vi "FPGA Main with speed output.vi"() -> ()   [LabVIEW 2018]
doc: "This VI reads all analogue data channels available at the fastest rate supported by the respective hardware and updates a memory address for when each measurement is available.\n\nAt a rate defined by the fastest module (NI 9237 - default of 12.5kHz) this memory is read, combined with the measurements from the 9237 module and written to the FIFO for communication to the RT machine.\n\nThe NI 9237 modeul therefore defines the nominal sampling rate of the system (with slower channels over-sampled).\n\nA time channel (in uSec) is provided with 0 referenced from the first acquisition of the NI 9237 module"
uses:
  <vilib>/LabVIEW Targets/FPGA/cRIO/shared/nicrio_ModuleControls/nicrio_cRIO-9237_DataRatesRing.ctl
  <vilib>/Platform/TimedLoop/XDataNode/timing_clust.ctl
  <vilib>/Platform/TimedLoop/XDataNode/nitl_modes.ctl
  <vilib>/Platform/TimedLoop/XDataNode/wakeup.ctl
  <vilib>/rvi/Emulation/niFpgaGetClockAttributes.vi
  <vilib>/rvi/Emulation/niFpgaSctlEmulationGetInTimedLoop.vi
  <vilib>/rvi/Emulation/niFpgaEmulationReportErrorSimple.vi
  <vilib>/rvi/Emulation/niFpgaProcessEmulError.vi
  <vilib>/rvi/eio/common/nirviEmuTemplatePropertySet_noerrors.vi
  <vilib>/rvi/eio/common/nirviEmuTemplateMethod_errors.vi
  <vilib>/rvi/interface/RandomDataEmulation/niFpgaRandomDataHandleErrors.vi
  <vilib>/rvi/Memory/Memory_Emulation/nirvimemoryFastEmulation.vi
  <vilib>/rvi/Memory/Memory_Emulation/nirvimemoryEmulation.vi
  <vilib>/rvi/Emulation/niFpgaEmulationIsFPGAContextNoSignature.vi
  <vilib>/rvi/DataTransferAndStorage/Container/Common/niFpgaContainerGetUniqueNameForEmu.vi
  <vilib>/rvi/errors/nirviReportUnexpectedCaseInternalError (U32).vi
  <vilib>/rvi/Emulation/niFpgaCriticalErrorInLSC.vi
  <vilib>/eio/EIOPropertyNode/EIOPropertyNode.xnode
  <vilib>/eio/EIONode/EIONode.xnode
  <vilib>/rvi/DataTransferAndStorage/Container/XNode/niFpgaContainer.xnode
  <vilib>/rvi/interface/RandomDataEmulation/nirviRandomDataFpgaReadWriteTemplate.vi
  <vilib>/platform/TimedLoop/XDataNode/XDataNode.xnode
  <vilib>/eio/EIOMethodNode/EIOMethodNode.xnode
  <vilib>/Platform/TimedLoop/XDataNode/XDNodeRunTimeDep.lvlib
  <vilib>/rvi/eio/common/nirviEmuTemplatePropertyGet_errors.vi
  <vilib>/rvi/eio/common/nirviEmuTemplatePropertyGet_noerrors.vi
  <vilib>/rvi/eio/common/nirviEmuTemplatePropertySet_errors.vi
panel:
  in  "speedOutputScaling":sgl=6366198.0
  in  "speedDirection":bool=TRUE
  in  "speed filter":u16=150
  in  "switch encoders":bool
  in  "falling edge (F)":bool caption="Torque encoder direction"
  in  "filterTorque":bool
  in  "Data Rate":T1=1 items=["50.000 kS/s (NI 9237)"=1, "25.000 kS/s (NI 9237)"=2, "16.667 kS/s (NI 9237)"=3, "12.500 kS/s (NI 9237)"=4, "10.000 kS/s (NI 9237)"=5, "8.333 kS/s (NI 9237)"=6, "7.143 kS/s (NI 9237)"=7, "6.250 kS/s (NI 9237)"=8, "5.556 kS/s (NI 9237)"=9, "5.000 kS/s (NI 9237)"=10, "4.545 kS/s (NI 9237)"=11, "4.167 kS/s (NI 9237)"=12, "3.846 kS/s (NI 9237)"=13, "3.571 kS/s (NI 9237)"=14, "3.333 kS/s (NI 9237)"=15, "3.125 kS/s (NI 9237)"=16, "2.941 kS/s (NI 9237)"=17, "2.778 kS/s (NI 9237)"=18, "2.632 kS/s (NI 9237)"=19, "2.500 kS/s (NI 9237)"=20, "2.381 kS/s (NI 9237)"=21, "2.273 kS/s (NI 9237)"=22, "2.174 kS/s (NI 9237)"=23, "2.083 kS/s (NI 9237)"=24, "2.000 kS/s (NI 9237)"=25, "1.923 kS/s (NI 9237)"=26, "1.852 kS/s (NI 9237)"=27, "1.786 kS/s (NI 9237)"=28, "1.724 kS/s (NI 9237)"=29, "1.667 kS/s (NI 9237)"=30, "1.613 kS/s (NI 9237)"=31]
  in  "encoders offset":sgl caption="encoder offset (radians)"
  out "Total channel count":u32=61
  out "timestamp":u32
  out "FIFO full counter":i32
  in  "Safe Voltage":fxp<+/-,20,5>[](array[numeric])=[0.0, 0.0, 0.0, 0.0]
  in  "Safe Digital":bool[](array[boolean])=[FALSE, FALSE, FALSE, FALSE, FALSE, FALSE, FALSE, FALSE]
  in  "Voltage Out":fxp<+/-,20,5>[](array[numeric])=[0.0, 0.0, 0.0, 0.0]
  in  "Update Outputs":bool
  in  "Mod 8":bool[](array[boolean])=[FALSE, FALSE, FALSE, FALSE, FALSE, FALSE, FALSE, FALSE]
  out "E Stop":bool
  in  "Stop acquire":bool
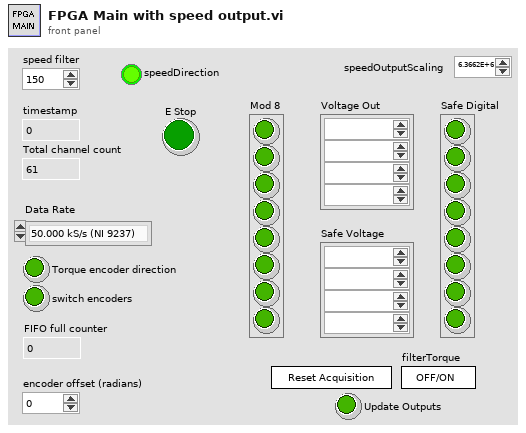
[diagram p1: front panel]
types:
  T1 = typedef "nicrio_cRIO-9237_DataRatesRing.ctl" = u8
  T2 = typedef "XDNodeRunTimeDep.lvlib/timing_clust.ctl" = cluster{"Expected End [f-1]":u64, "Actual End [f-1]":u64, "Finished Late? [f-1]":bool, "Expected End [i-1]":u64, "Actual End [i-1]":u64, "Finished Late? [i-1]":bool, "Expected Start [i]":u64, "Actual Start [i]":u64, "Expected Start [f]":u64, "Actual Start [f]":u64, "Source Name":string, "Structure Name":string, "Period":i64, "Deadline":i64, "Offset":i64, "Start":i64, "Priority":i32, "Timeout":i32, "Mode":T3, "Wakeup Reason":T4, "Error":errorcluster, "Source Type":string, "Secondary Source Type":string, "Global End Time":u64, "Global Start Time":u64, "Frame Duration":u64, "Iteration Duration":u64, "Assigned CPU":i32, "I/O Scan Engine Mode":u32}
  T3 = typedef "XDNodeRunTimeDep.lvlib/nitl_modes.ctl" = enum32{"No Change", "Process missed periods, maintain original phase", "Discard missed periods, maintain original phase", "Process missed periods, ignore original phase", "Discard missed periods, ignore original phase"}
  T4 = typedef "XDNodeRunTimeDep.lvlib/wakeup.ctl" = enum32{"Normal", "Aborted", "Asynchronous wakeup", "Timing source error", "Timed loop error", "Timeout"}
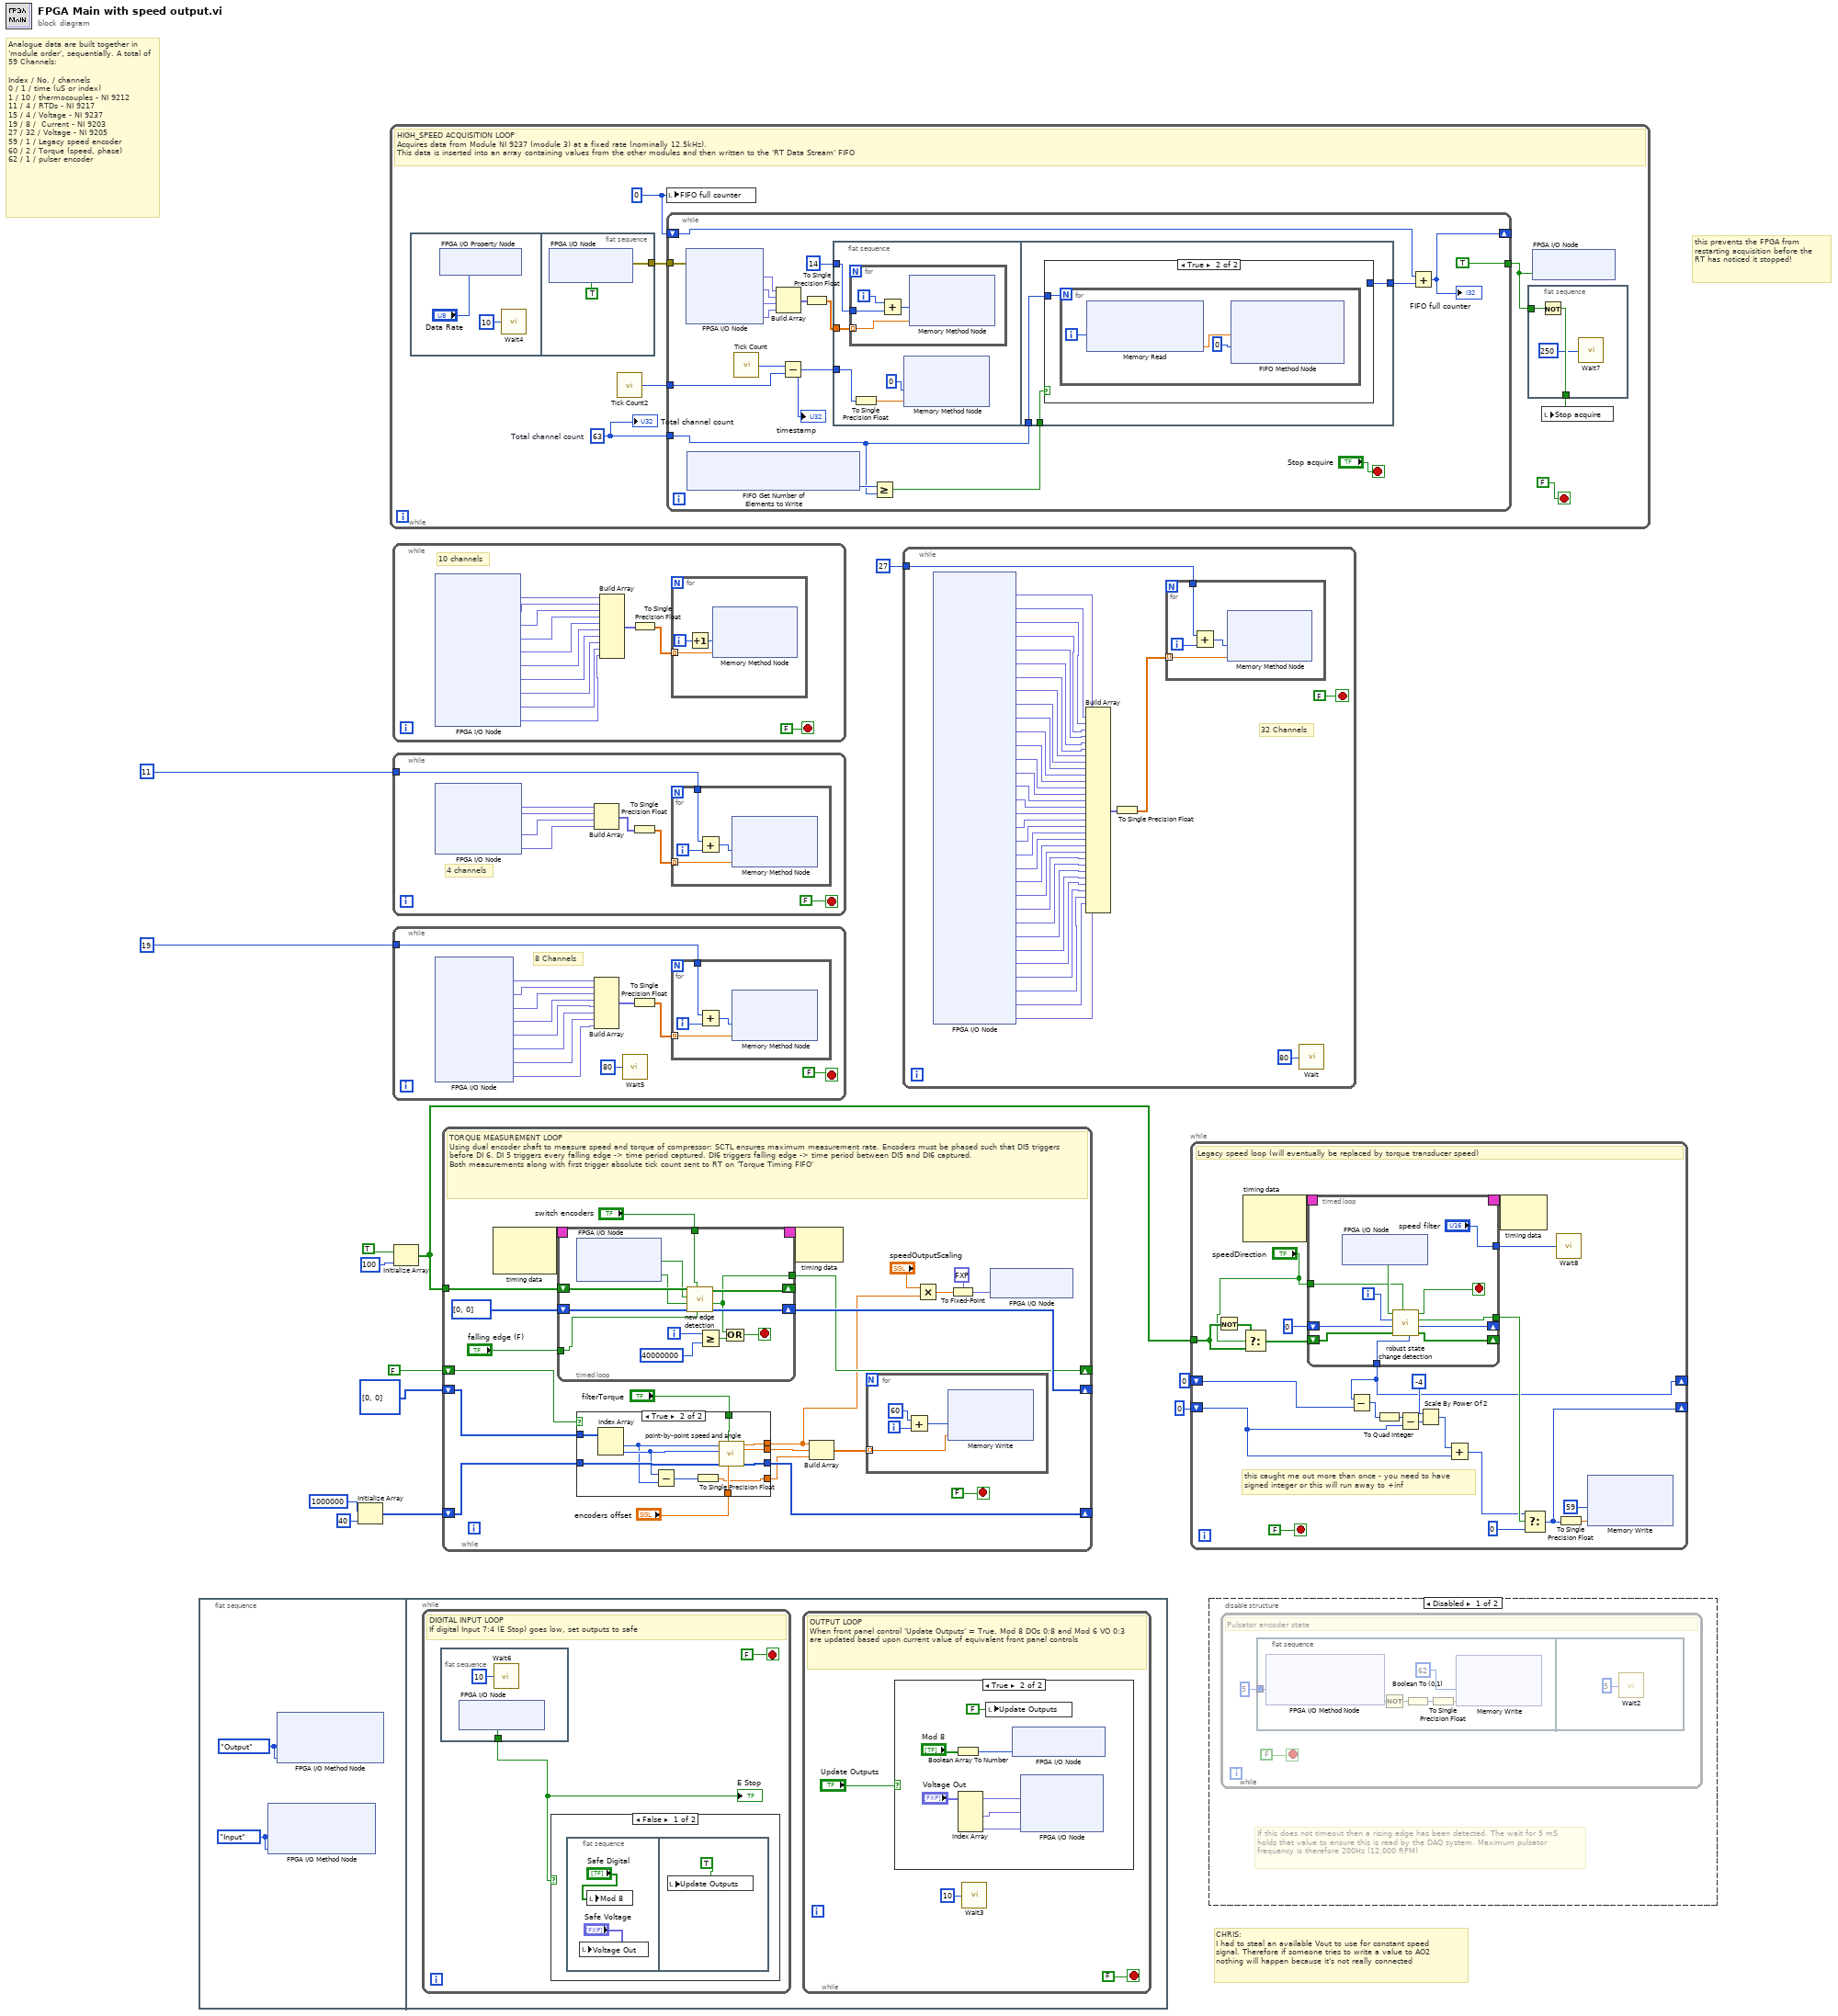
[diagram p0: block diagram]
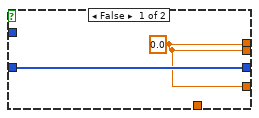
[diagram p5: hidden frame]
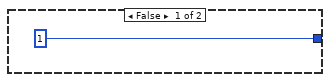
[diagram p6: hidden frame]
diagram:
  # "CHRIS:\nI had to steal an available Vout to use for constant speed signal. Therefore if someone tries to write a value to AO2 nothing will happen because it's not really connected"
  # "this prevents the FPGA from restarting acquisition before the RT has noticed it stopped!"
  # "Analogue data are built together in 'module order', sequentially. A total of 59 Channels:\n\nIndex / No. / channels\n0 / 1 / time (uS or index)\n1 / 10 / thermocouples - NI 9212\n11 / 4 / RTDs - NI 9217\n15 / 4 / Voltage - NI 9237\n19 / 8 /  Current - NI 9203\n27 / 32 / Voltage - NI 9205\n59 / 1 / Legacy speed encoder\n60 / 2 / Torque (speed, phase)\n62 / 1 / pulser encoder"
  n1 = flat-sequence {
    frame #0 {
      w14 = enum8{"No Change", "Input", "Output"}."Output" ("DIO 7:4")
      w15 = enum8{"No Change", "Input", "Output"}."Input" ("DIO 7:4")
      n2 = xnode "FPGA I/O Method Node"("DIO 7:4"=w15, "DIO 3:0"=w15) -> ()  [unwired: 1 in, 1 out]
      n3 = xnode "FPGA I/O Method Node"("DIO 7:4"=w14, "DIO 3:0"=w14) -> ()  [unwired: 1 in, 1 out]
    }
    frame #1 {
      n4 = while {
        stop <- FALSE stop-if-true
        # "DIGITAL INPUT LOOP\nIf digital Input 7:4 (E Stop) goes low, set outputs to safe"
        n5 = flat-sequence {
          tunnel: [w29] -> w26
          frame #0 {
            n6 = xnode "FPGA I/O Node"() -> ("Mod7/DIO4"=w29:bool)  [unwired: 1 in, 1 out]
            n7 = call "Wait6"("Count(uSec)"=u8 10) -> ()  [unwired: 1 out]
          }
        }
        n8 = case shown="False" w26 {
          frame False {
            n9 = flat-sequence {
              frame #0 {
                n10 = local write "Voltage Out"("Safe Voltage") -> ()
                n11 = local write "Mod 8"("Safe Digital") -> ()
              }
              frame #1 {
                n12 = local write "Update Outputs"(TRUE ("Update Outputs")) -> ()
              }
            }
          }
          frame True {
          }
        }
        "E Stop" <- w26
      }
      n13 = while {
        stop <- FALSE stop-if-true
        # "OUTPUT LOOP\nWhen front panel control 'Update Outputs' = True, Mod 8 DOs 0:8 and Mod 6 VO 0:3 are updated based upon current value of equivalent front panel controls"
        n14 = case shown="True" "Update Outputs" {
          frame False {
          }
          frame True {
            n15 = Boolean Array To Number(Boolean array="Mod 8") -> (number=w24:u8)
            n16 = Index Array(array="Voltage Out") -> (element #1=w22:fxp<+/-,20,5>, element #2=w21:fxp<+/-,20,5>, element #4=w19:fxp<+/-,20,5>)  [unwired: 4 in, 1 out]
            n17 = local write "Update Outputs"(FALSE ("Update Outputs")) -> ()
            n18 = xnode "FPGA I/O Node"("Mod8/DIO7:0"=w24) -> ()  [unwired: 1 in, 1 out]
            n19 = xnode "FPGA I/O Node"("Mod6/AO0"=w22, "Mod6/AO1"=w21, "Mod6/AO3"=w19) -> ()  [unwired: 3 in, 3 out]
          }
        }
        n20 = call "Wait3"("Count(uSec)"=u16 10 ("Count(Ticks)")) -> ()  [unwired: 1 out]
      }
    }
  }
  n21 = Initialize Array(u32 1000000 ("64bit integer"), 40 ("dimension size")) -> (w8:u32[])
  n22 = while {
    stop <- FALSE stop-if-true
    w34 = 0 ("FIFO full counter")
    w37 = u32 63  # Total channel count
    # "HIGH_SPEED ACQUISITION LOOP\nAcquires data from Module NI 9237 (module 3) at a fixed rate (nominally 12.5kHz).\nThis data is inserted into an array containing values from the other modules and then written to the 'RT Data Stream' FIFO"
    n23 = flat-sequence {
      tunnel: [w46] -> w38
      frame #0 {
        n24 = xnode "FPGA I/O Property Node"("Data Rate"="Data Rate") -> ()  [unwired: 1 in, 1 out]
        n25 = call "Wait4"("Count(mSec)"=u16 10) -> ()  [unwired: 1 out]
      }
      frame #1 {
        n26 = xnode "FPGA I/O Node"("Mod3/Start"=TRUE) -> ("error out"=w46:errorcluster)  [unwired: 2 in, 1 out]
      }
    }
    n27 = call "Tick Count2"() -> ("Tick Count(uSec)"=w39:u32)
    n28 = local write "FIFO full counter"(w34) -> ()
    n29 = while {
      tunnel: [TRUE ("I/O Item")] -> w36
      tunnel: w38 -> [w64]
      tunnel: w37 -> [w49]
      shift-right: [w57] -> _
      shift-left: w34 -> [w55]
      tunnel: w39 -> [w58]
      stop <- "Stop acquire" stop-if-true
      n30 = xnode "FPGA I/O Node"("error in"=w64) -> ("Mod3/AI0"=w63:fxp<+/-,24,-4>, "Mod3/AI1"=w62:fxp<+/-,24,-4>, "Mod3/AI2"=w61:fxp<+/-,24,-4>, "Mod3/AI3"=w60:fxp<+/-,24,-4>)  [unwired: 4 in, 5 out]
      n31 = xnode ("FIFO Get Number of Elements to Write")() -> ("Number of Elements to Write"=w51:u32)  [unwired: 1 in, 1 out]
      n32 = call "Tick Count"() -> ("Tick Count(uSec)"=w54:u32)
      n33 = Build Array(w63, w62, w61, w60) -> (w59:fxp<+/-,24,-4>[])
      n34 = Subtract(x=w54, y=w58) -> (x-y=w47:u32)
      "timestamp" <- w47
      n35 = To Single Precision Float(number=w59) -> (single precision float=w53:sgl[])
      n36 = flat-sequence {
        tunnel: w53 -> [w70]
        tunnel: 14 ("index") -> [w69]
        tunnel: w47 -> [w67]
        tunnel: w49 -> [w77]
        tunnel: [w76] -> w48
        tunnel: w50 -> [w75]
        frame #0 {
          n37 = for {
            tunnel: w70 -> [w74] mode=indexing
            tunnel: w69 -> [w73]
            i -> [w71]
            n38 = Add(x=w71, y=w73) -> (x+y=w72:i32)
            n39 = xnode ("Memory Method Node")("Address"=w72, "Data"=w74) -> ()  [unwired: 1 in, 1 out]
          }
          n40 = To Single Precision Float(number=w67) -> (single precision float=w68:sgl)
          n41 = xnode ("Memory Method Node")("Address"=u32 0, "Data"=w68) -> ()  [unwired: 1 in, 1 out]
        }
        frame #1 {
          n42 = case shown="True" w75 {
            tunnel: [1 _] -> w76
            tunnel: w77 -> [_ w79]
            frame False {
            }
            frame True {
              n43 = for {
                N: w79 -> [_]
                i -> [w80]
                n44 = xnode ("Memory Read")("Address"=w80) -> ("Data"=w81:sgl)  [unwired: 1 in, 1 out]
                n45 = xnode ("FIFO Method Node")("Element"=w81, "Timeout"=0) -> ()  [unwired: 1 in, 2 out]
              }
            }
          }
        }
      }
      n46 = Greater Or Equal?(x=w51, y=w49) -> (x >= y?=w50:bool)
      n47 = Add(x=w55, y=w48) -> (x+y=w57:i32)
      "FIFO full counter" <- w57
    }
    n48 = flat-sequence {
      tunnel: w36 -> [w42]
      tunnel: [w41] -> w33
      frame #0 {
        n49 = Not(x=w42) -> (.not. x?=w41:bool)
        n50 = call "Wait7"("Count(mSec)"=u8 250) -> ()  [unwired: 1 out]
      }
    }
    n51 = xnode "FPGA I/O Node"("Mod3/Stop"=w36) -> ()  [unwired: 1 in, 1 out]
    n52 = local write "Stop acquire"(w33) -> ()
    "Total channel count" <- w37
  }
  n53 = while {
    stop <- FALSE stop-if-true
    # "10 channels"
    n54 = xnode "FPGA I/O Node"() -> ("Mod1/TC0"=w95:fxp<+/-,24,-2>, "Mod1/TC1"=w94:fxp<+/-,24,-2>, "Mod1/TC2"=w93:fxp<+/-,24,-2>, "Mod1/TC3"=w92:fxp<+/-,24,-2>, "Mod1/TC4"=w91:fxp<+/-,24,-2>, "Mod1/TC5"=w90:fxp<+/-,24,-2>, "Mod1/TC6"=w89:fxp<+/-,24,-2>, "Mod1/TC7"=w88:fxp<+/-,24,-2>, "Mod1/CJC0"=w85:fxp<+/-,24,-2>, "Mod1/CJC1"=w84:fxp<+/-,24,-2>)  [unwired: 10 in, 10 out]
    n55 = Build Array(w95, w94, w93, w92, w91, w90, w89, w88, w85, w84) -> (w87:fxp<+/-,24,-2>[])
    n56 = To Single Precision Float(number=w87) -> (single precision float=w86:sgl[])
    n57 = for {
      tunnel: w86 -> [w98] mode=indexing
      i -> [w97]
      n58 = Increment(x=w97) -> (x+1=w96:i32)
      n59 = xnode ("Memory Method Node")("Address"=w96, "Data"=w98) -> ()  [unwired: 1 in, 1 out]
    }
  }
  n60 = while {
    tunnel: 11 ("Numeric") -> [w100]
    stop <- FALSE stop-if-true
    # "4 channels"
    n61 = xnode "FPGA I/O Node"() -> ("Mod2/RTD0"=w106:fxp<+/-,24,10>, "Mod2/RTD1"=w105:fxp<+/-,24,10>, "Mod2/RTD2"=w104:fxp<+/-,24,10>, "Mod2/RTD3"=w101:fxp<+/-,24,10>)  [unwired: 4 in, 4 out]
    n62 = Build Array(w106, w105, w104, w101) -> (w103:fxp<+/-,24,10>[])
    n63 = To Single Precision Float(number=w103) -> (single precision float=w102:sgl[])
    n64 = for {
      tunnel: w102 -> [w110] mode=indexing
      tunnel: w100 -> [w107]
      i -> [w109]
      n65 = Add(x=w107, y=w109) -> (x+y=w108:i32)
      n66 = xnode ("Memory Method Node")("Address"=w108, "Data"=w110) -> ()  [unwired: 1 in, 1 out]
    }
  }
  n67 = while {
    tunnel: 19 ("Numeric") -> [w117]
    stop <- FALSE stop-if-true
    # "8 Channels"
    n68 = xnode "FPGA I/O Node"() -> ("Mod4/AI0"=w123:fxp<+/-,21,-4>, "Mod4/AI1"=w122:fxp<+/-,21,-4>, "Mod4/AI2"=w121:fxp<+/-,21,-4>, "Mod4/AI3"=w118:fxp<+/-,21,-4>, "Mod4/AI4"=w116:fxp<+/-,21,-4>, "Mod4/AI5"=w115:fxp<+/-,21,-4>, "Mod4/AI6"=w114:fxp<+/-,21,-4>, "Mod4/AI7"=w113:fxp<+/-,21,-4>)  [unwired: 8 in, 8 out]
    n69 = Build Array(w123, w122, w121, w118, w116, w115, w114, w113) -> (w120:fxp<+/-,21,-4>[])
    n70 = call "Wait5"("Count(uSec)"=u8 80) -> ()  [unwired: 1 out]
    n71 = To Single Precision Float(number=w120) -> (single precision float=w119:sgl[])
    n72 = for {
      tunnel: w119 -> [w127] mode=indexing
      tunnel: w117 -> [w124]
      i -> [w126]
      n73 = Add(x=w124, y=w126) -> (x+y=w125:i32)
      n74 = xnode ("Memory Method Node")("Address"=w125, "Data"=w127) -> ()  [unwired: 1 in, 1 out]
    }
  }
  n75 = Initialize Array(TRUE, 100 ("edge buffer size")) -> (w4:bool[])
  n76 = while {
    shift-right: [w148] -> _
    shift-left: w8 -> [w149]
    tunnel: w4 -> [w147]
    shift-right: [w136] -> _
    shift-left: u32[] [0, 0] ("step") -> [w135]
    shift-right: [w133] -> _
    shift-left: FALSE ("edge detected") -> [w134]
    stop <- FALSE stop-if-true
    # "TORQUE MEASUREMENT LOOP\nUsing dual encoder shaft to measure speed and torque of compressor: SCTL ensures maximum measurement rate. Encoders must be phased such that DI5 triggers before DI 6. DI 5 triggers every falling edge -> time period captured. DI6 triggers falling edge -> time period between DI5 and DI6 captured.\nBoth measurements along with first trigger absolute tick count sent to RT on 'Torque Timing FIFO'"
    n77 = node-c288() -> (w145:T2)  [unwired: 2 in]
    n78 = timed-loop {
      timing: w145 -> [_]
      timing-out: [_] -> w144
      shift-right: [w174] -> _
      shift-left: w147 -> [w177]
      shift-right: [w175] -> w136
      shift-left: u32[] [0, 0] ("step") -> [w176]
      tunnel: "falling edge (F)" -> [w171]
      tunnel: [w172] -> w133
      tunnel: "switch encoders" -> [w168]
      i -> [w180]
      stop <- w173 stop-if-true
      n79 = xnode "FPGA I/O Node"() -> ("Mod7/DIO0"=w170:bool, "Mod7/DIO1"=w169:bool)  [unwired: 2 in, 2 out]
      n80 = call "new edge detection.vi"("rising edge (T)"=w171, "switch encoders (F)"=w168, "ticks"=w176, "encoder 2"=w169, "encoder 1"=w170, "history in"=w177) -> ("ticks out"=w175:u32[], "edge detected"=w172:bool, "history out"=w174:bool[])  [unwired: 3 in]
      n81 = Greater Or Equal?(x=w180, y=40000000) -> (x >= y?=w178:bool)
      n82 = Or(x=w172, y=w178) -> (x .or. y?=w173:bool)
    }
    n83 = case shown="True" w134 {
      tunnel: w149 -> [w152 w163]
      tunnel: [w152 w162] -> w148
      tunnel: [w151 w161] -> w132
      tunnel: [w151 w160] -> w138
      tunnel: w135 -> [_ w159]
      tunnel: "encoders offset" -> [_ w158]
      tunnel: "filterTorque" -> [_ w157]
      tunnel: [w151 w153] -> w137
      frame False {
        w151 = sgl 0.0 ("calculated speed (Hz)")
      }
      frame True {
        n84 = Index Array(array=w159) -> (element #1=w155:u32, element #2=w156:u32)  [unwired: 2 in]
        n85 = Subtract(x=w156, y=w155) -> (x-y=w154:u32)
        n86 = To Single Precision Float(number=w154) -> (single precision float=w153:sgl)
        n87 = call "point-by-point speed and angle.vi"("encoder fixed offest"=w158, "filter torque"=w157, "speed history in"=w163, "angle pulse"=w156, "speed pulse"=w155) -> ("speed history out"=w162:u32[], "calculated angle (radians)"=w160:sgl, "calculated speed (rad/tick)"=w161:sgl)  [unwired: 4 in]
      }
    }
    n88 = node-c288(w144) -> ()  [unwired: 1 out]
    n89 = Build Array(w132, w138, w137) -> (w141:sgl[])
    n90 = for {
      tunnel: w141 -> [w164] mode=indexing
      i -> [w165]
      n91 = Add(x=u32 60 ("Address"), y=w165) -> (x+y=w166:u32)
      n92 = xnode ("Memory Write")("Address"=w166, "Data"=w164) -> ()  [unwired: 1 in, 1 out]
    }
    n93 = Multiply(x="speedOutputScaling", y=w132) -> (x*y=w130:sgl)
    n94 = To Fixed-Point(fixed-point type=fxp<+/-,20,5> 0.0 ("Mod6/AO2"), number=w130) -> (fixed-point=w129:fxp<+/-,20,5>)
    n95 = xnode "FPGA I/O Node"("Mod6/AO2"=w129) -> ()  [unwired: 1 in, 1 out]
  }
  n96 = while {
    tunnel: 27 ("Numeric") -> [w220]
    stop <- FALSE stop-if-true
    # "32 Channels"
    n97 = xnode "FPGA I/O Node"() -> ("Mod5/AI0"=w188:fxp<+/-,26,5>, "Mod5/AI1"=w189:fxp<+/-,26,5>, "Mod5/AI2"=w190:fxp<+/-,26,5>, "Mod5/AI3"=w191:fxp<+/-,26,5>, "Mod5/AI4"=w192:fxp<+/-,26,5>, "Mod5/AI5"=w193:fxp<+/-,26,5>, "Mod5/AI6"=w194:fxp<+/-,26,5>, "Mod5/AI7"=w195:fxp<+/-,26,5>, "Mod5/AI8"=w219:fxp<+/-,26,5>, "Mod5/AI9"=w218:fxp<+/-,26,5>, "Mod5/AI10"=w217:fxp<+/-,26,5>, "Mod5/AI11"=w216:fxp<+/-,26,5>, "Mod5/AI12"=w215:fxp<+/-,26,5>, "Mod5/AI13"=w214:fxp<+/-,26,5>, "Mod5/AI14"=w213:fxp<+/-,26,5>, "Mod5/AI15"=w212:fxp<+/-,26,5>, "Mod5/AI16"=w211:fxp<+/-,26,5>, "Mod5/AI17"=w210:fxp<+/-,26,5>, "Mod5/AI18"=w209:fxp<+/-,26,5>, "Mod5/AI19"=w208:fxp<+/-,26,5>, "Mod5/AI20"=w207:fxp<+/-,26,5>, "Mod5/AI21"=w206:fxp<+/-,26,5>, "Mod5/AI22"=w205:fxp<+/-,26,5>, "Mod5/AI23"=w204:fxp<+/-,26,5>, "Mod5/AI24"=w203:fxp<+/-,26,5>, "Mod5/AI25"=w202:fxp<+/-,26,5>, "Mod5/AI26"=w201:fxp<+/-,26,5>, "Mod5/AI27"=w200:fxp<+/-,26,5>, "Mod5/AI28"=w199:fxp<+/-,26,5>, "Mod5/AI29"=w198:fxp<+/-,26,5>, "Mod5/AI30"=w197:fxp<+/-,26,5>, "Mod5/AI31"=w196:fxp<+/-,26,5>)  [unwired: 32 in, 32 out]
    n98 = Build Array(w188, w189, w190, w191, w192, w193, w194, w195, w219, w218, w217, w216, w215, w214, w213, w212, w211, w210, w209, w208, w207, w206, w205, w204, w203, w202, w201, w200, w199, w198, w197, w196) -> (w221:fxp<+/-,26,5>[])
    n99 = To Single Precision Float(number=w221) -> (single precision float=w187:sgl[])
    n100 = for {
      tunnel: w187 -> [w225] mode=indexing
      tunnel: w220 -> [w222]
      i -> [w224]
      n101 = Add(x=w222, y=w224) -> (x+y=w223:i32)
      n102 = xnode ("Memory Method Node")("Address"=w223, "Data"=w225) -> ()  [unwired: 1 in, 1 out]
    }
    n103 = call "Wait"("Count(uSec)"=u8 80) -> ()  [unwired: 1 out]
  }
  n104 = while {
    shift-right: [w236] -> _
    shift-left: i64 0 -> [w242]
    tunnel: w4 -> [w228]
    shift-right: [w232] -> _
    shift-left: u32 0 ("tick") -> [w231]
    stop <- FALSE stop-if-true
    # "this caught me out more than once - you need to have signed integer or this will run away to +inf"
    # "Legacy speed loop (will eventually be replaced by torque transducer speed)"
    n105 = Not(x=w228) -> (.not. x?=w229:bool[])
    n106 = node-c288() -> (w248:T2)  [unwired: 2 in]
    n107 = Select(t=w229, s="speedDirection", f=w228) -> (s? t:f=w227:bool[])
    n108 = timed-loop {
      timing: w248 -> [_]
      timing-out: [_] -> w247
      shift-right: [w256] -> _
      shift-left: i16 0 ("step") -> [w257]
      tunnel: [w254] -> w237
      tunnel: [w253] -> w232
      shift-right: [w251] -> _
      shift-left: w227 -> [w252]
      tunnel: ["speed filter"] -> w230
      tunnel: "speedDirection" -> [w249]
      i -> [w258]
      stop <- w255 stop-if-true
      n109 = xnode "FPGA I/O Node"() -> ("Mod7/DIO3"=w259:bool)  [unwired: 1 in, 1 out]
      n110 = call "robust state change detection.vi"("falling edge (F)"=w249, "history"=w252, "step"=w257, "tick"=w258, "New state"=w259) -> ("history out"=w251:bool[], "step out"=w256:i16, "edge detected"=w254:bool, "Stop?"=w255:bool, "tick"=w253:u32)  [unwired: 2 in]
    }
    n111 = Subtract(x=w232, y=w231) -> (x-y=w233:u32)
    n112 = To Quad Integer(1:w233) -> (0:w239:i64)
    n113 = Subtract(x=w239, y=w242) -> (x-y=w243:i64)
    n114 = Scale By Power Of 2(n=i16 -4, x=w243) -> (x*2^n=w245:i64)
    n115 = Add(x=w245, y=w242) -> (x+y=w234:i64)
    n116 = node-c288(w247) -> ()  [unwired: 1 out]
    n117 = Select(t=w234, s=w237, f=u32 0 ("t")) -> (s? t:f=w236:i64)
    n118 = call "Wait8"("Count(uSec)"=w230) -> ()  [unwired: 1 out]
    n119 = To Single Precision Float(number=w236) -> (single precision float=w241:sgl)
    n120 = xnode ("Memory Write")("Address"=u32 59, "Data"=w241) -> ()  [unwired: 1 in, 1 out]
  }
  n121 = disable-structure shown="Disabled" {
    frame Disabled {
      # "If this does not timeout then a rising edge has been detected. The wait for 5 mS holds that value to ensure this is read by the DAQ system. Maximum pulsator frequency is therefore 200Hz (12,000 RPM)"
      n122 = while {
        stop <- FALSE stop-if-true
        # "Pulsator encoder state"
        n123 = flat-sequence {
          tunnel: 5 ("Timeout") -> [w268]
          frame #0 {
            n124 = xnode "FPGA I/O Method Node"("Timeout"=w268) -> ("Timed Out"=w267:bool)  [unwired: 1 in, 1 out]
            n125 = Not(x=w267) -> (.not. x?=w266:bool)
            n126 = Boolean To (0,1)(Boolean=w266) -> (0, 1=w271:i16)
            n127 = To Single Precision Float(number=w271) -> (single precision float=w270:sgl)
            n128 = xnode ("Memory Write")("Address"=u32 62, "Data"=w270) -> ()  [unwired: 1 in, 1 out]
          }
          frame #1 {
            n129 = call "Wait2"("Count(mSec)"=u16 5 ("Count(uSec)")) -> ()  [unwired: 1 out]
          }
        }
      }
    }
    frame Enabled {
    }
  }
